vi "cfc_center.vi"(0 "Fitted Pos":dbl[](array[numeric]), 2 "Nb pts X&Y":u32, 3 "X_cfc":dbl, 5 "Y_cfc":dbl) -> (6 "X volt":dbl, 7 "Y volt":dbl, 8 "Intensity":dbl)   [LabVIEW 2015]
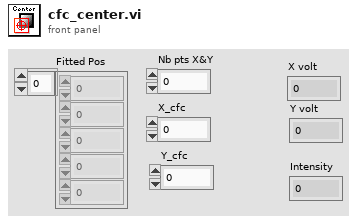
[diagram p1: front panel]
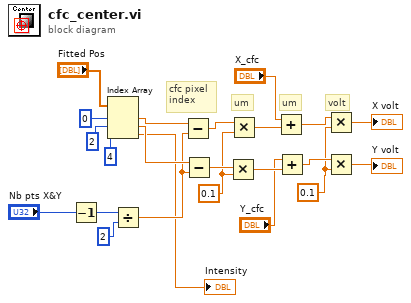
[diagram p0: block diagram]
diagram:
  w4 = 0.1 ("y")
  w11 = 0.1 ("y")
  # "volt"
  # "um"
  # "um"
  # "cfc pixel \nindex"
  n1 = Decrement(x="Nb pts X&Y") -> (x-1=w17:u32)
  n2 = Index Array(array="Fitted Pos", index #1=0 ("index"), index #2=2 ("index"), index #3=4 ("index")) -> (element #1=w19:dbl, element #2=w18:dbl, element #3=→"Intensity":dbl)
  n3 = Divide(x=w17, y=u32 2) -> (x/y=w14:dbl)
  n4 = Subtract(x=w19, y=w14) -> (x-y=w13:dbl)
  n5 = Subtract(x=w18, y=w14) -> (x-y=w12:dbl)
  n6 = Multiply(x=w12, y=w11) -> (x*y=w9:dbl)
  n7 = Multiply(x=w13, y=w11) -> (x*y=w10:dbl)
  n8 = Add(x="X_cfc", y=w10) -> (x+y=w5:dbl)
  n9 = Add(x="Y_cfc", y=w9) -> (x+y=w6:dbl)
  n10 = Multiply(x=w5, y=w4) -> (x*y=→"X volt":dbl)
  n11 = Multiply(x=w6, y=w4) -> (x*y=→"Y volt":dbl)
